vi "Get Coverage for VI.vi"(8 "error in (no error)":errorcluster, 10 "VI Path":path, 11 "Coverage Analyzer in":refnum<class "Coverage Analyzer.lvclass">) -> (0 "error out":errorcluster, 1 "Coverage Measured?":bool, 2 "Percentage":dbl, 3 "Coverage Analyzer out":refnum<class "Coverage Analyzer.lvclass">)   [LabVIEW 2020, in "Coverage Analyzer.lvclass"]
uses:
  Coverage Analyzer.lvclass
  Coverage Analyzer.lvclass/Coverage Analyzer.ctl
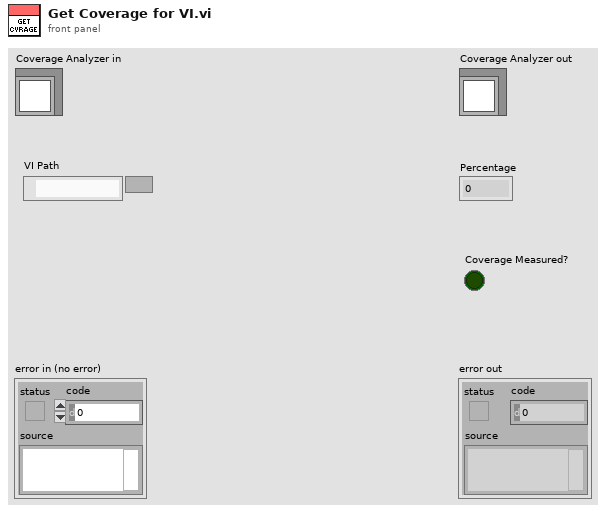
[diagram p1: front panel]
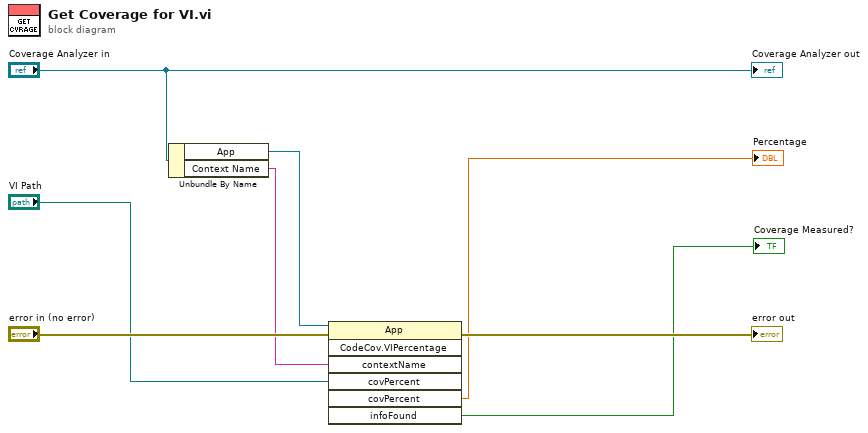
[diagram p0: block diagram]
diagram:
  n1 = Unbundle By Name("Coverage Analyzer in") -> ("App"=w5:refnum<vi>, "Context Name"=w3:string)
  n2 = invoke class="App" method="CodeCov.VIPercentage"(reference=w5, error in="error in (no error)", "contextName"=w3, "covPercent"="VI Path") -> (error out=→"error out":errorcluster, "covPercent"=→"Percentage":dbl, "infoFound"=→"Coverage Measured?":bool)  [unwired: 3 in, 4 out]
  "Coverage Analyzer out" <- "Coverage Analyzer in"
